vi "Resample (constant to variable,single-channel).vi"(5 "anti-aliasing?":bool=TRUE, 6 "FIR filter specifications":T1={"alias rejection (dB)"=120.0, "normalized bandwidth"=0.4536} {"normalized bandwidth" format="%.4f"; "alias rejection (dB)" format="%.2f"}, 7 "reset?":bool, 8 "error in (no error)":errorcluster, 10 "Time":dbl[](array[numeric]), 11 "X":dbl[](array[numeric])) -> (0 "error out":errorcluster, 2 "Time Stamps":dbl[](array[numeric]) format="%#.6g", 3 "Y":dbl[](array[numeric]))   [LabVIEW 2014, in "NI_AALPro.lvlib"]
doc: "Resamples input signal <B>X</B> according to <B>Time</B> using an FIR filter implementation. Wire data to the <B>X</B> input to determine the polymorphic instance to use or manually select the instance."
uses:
  NI_AALPro.lvlib
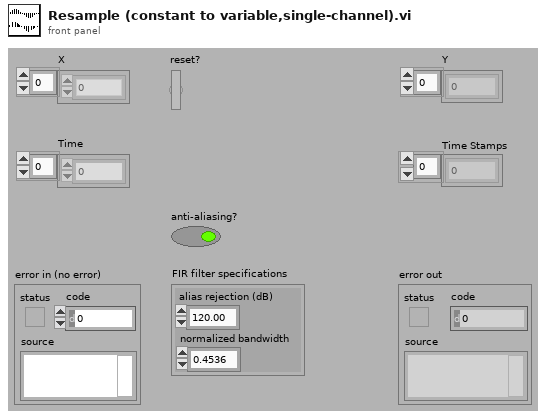
[diagram p1: front panel]
types:
  T1 = cluster{"alias rejection (dB)":dbl, "normalized bandwidth":dbl}
  T2 = cluster{"status":bool, "time not in ascending order":i32, "source":string}
  T3 = cluster{"timing jitter":enum32{"Interpolation", "Rounding"}, "anti-aliasing?":bool, "filter prototype":cluster{"coefficients":dbl[], "factor":i32}}
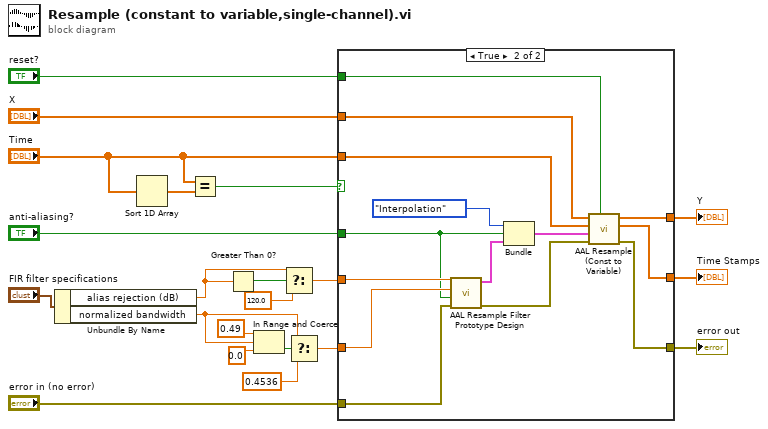
[diagram p0: block diagram]
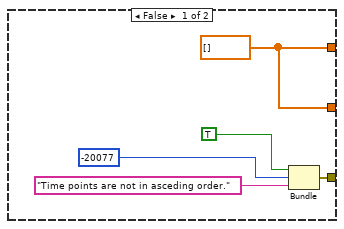
[diagram p2: hidden frame]
diagram:
  n1 = Unbundle By Name("FIR filter specifications") -> ("alias rejection (dB)"=w2:dbl, "normalized bandwidth"=w5:dbl)
  n2 = Sort 1D Array(array="Time") -> (sorted array=w14:dbl[])
  n3 = Equal?(x="Time", y=w14) -> (x = y?=w12:bool)
  n4 = Greater Than 0?(x=w2) -> (x > 0?=w1:bool)
  n5 = In Range and Coerce(upper limit=0.49, x=w5, lower limit=0.0 ("upper limit")) -> (In Range?=w7:bool)  [unwired: 1 out]
  n6 = Select(t=w2, s=w1, f=120.0) -> (s? t:f=w4:dbl)
  n7 = Select(t=w5, s=w7, f=0.4536 ("upper limit")) -> (s? t:f=w3:dbl)
  n8 = case shown="True" w12 {
    tunnel: "anti-aliasing?" -> [_ w27]
    tunnel: "Time" -> [_ w36]
    tunnel: [w26 w35] -> w20
    tunnel: [w22 w34] -> w19
    tunnel: "reset?" -> [_ w33]
    tunnel: "X" -> [_ w32]
    tunnel: [w26 w31] -> w16
    tunnel: "error in (no error)" -> [_ w30]
    tunnel: w4 -> [_ w29]
    tunnel: w3 -> [_ w28]
    frame False {
      w26 = dbl[] [] ("Y")
      n9 = Bundle("status"=TRUE, "time not in ascending order"=-20077, "source"="Time points are not in asceding order.") -> (w22:T2)  [unwired: 1 in]
    }
    frame True {
      n10 = call "AAL Resample Filter Prototype Design.vi"("error in (no error)"=w30, "alias free"=w27, "normalized bandwidth"=w28, "A stop [dB]"=w29) -> ("error out"=w40:errorcluster, "filter prototype"=w38:cluster{"coefficients":dbl[], "factor":i32})  [unwired: 5 in, 1 out]
      n11 = Bundle("timing jitter"=enum32{"Interpolation", "Rounding"}."Interpolation", "anti-aliasing?"=w27, "filter prototype"=w38) -> (w37:T3)  [unwired: 1 in]
      n12 = call "AAL Resample (Const to Variable).vi"("reset? (True)"=w33, "error in (no error)"=w40, "config"=w37, "time"=w36, "X"=w32) -> ("error out"=w34:errorcluster, "time stamps"=w31:dbl[], "Y"=w35:dbl[])  [unwired: 3 in, 1 out]
    }
  }
  "error out" <- w19
  "Y" <- w20
  "Time Stamps" <- w16
